vi "Start.vi"(1 "Graph refs":T2, 2 "Delays refs":T5, 6 "buttons refs":T4, 8 "error in (no error)":errorcluster, 9 "Slider cluster":T6, 10 "extra refs":T1, 11 "Control-Client in":refnum<class "Control-Client.lvclass">) -> (0 "error out":errorcluster, 3 "Control-Client out":refnum<class "Control-Client.lvclass">, 4 "Cells pos":dbl[](array[numeric]), 5 "ControlEventCom event":refnum<event-registration>)   [LabVIEW 2015, in "Control-Client.lvclass"]
uses:
  Control-Client.lvclass
  dependecies/ControlsVIs/Clusters-def/Delays-refs_CLIENT.ctl
  dependecies/ControlsVIs/Clusters-def/Controls-with-permissions_CLIENT.ctl
  controls/DigitalIndicatorELYSEpulses.ctl
  controls/CellsSD.ctl
  controls/CellBoolean.ctl
  dependecies/XControls/CellsDL/ControlDL.xctl
  controls/Gauge_pump/Gauge_pump.xctl
  controls/WCM.ctl
  dependecies/ControlsVIs/Clusters-def/Graphs_ref_Client.ctl
  dependecies/ControlsVIs/Clusters-def/graphs_TR.ctl
  dependecies/ControlsVIs/Clusters-def/Message types.ctl
  Control-Client.lvclass/Control-Client.ctl
  GeneralFunctionality/GeneralFunctionality.lvclass/GeneralFunctionality.ctl
  Message/Message.lvclass/Message.ctl
  Message/Message.lvclass
  GeneralFunctionality/GeneralFunctionality.lvclass
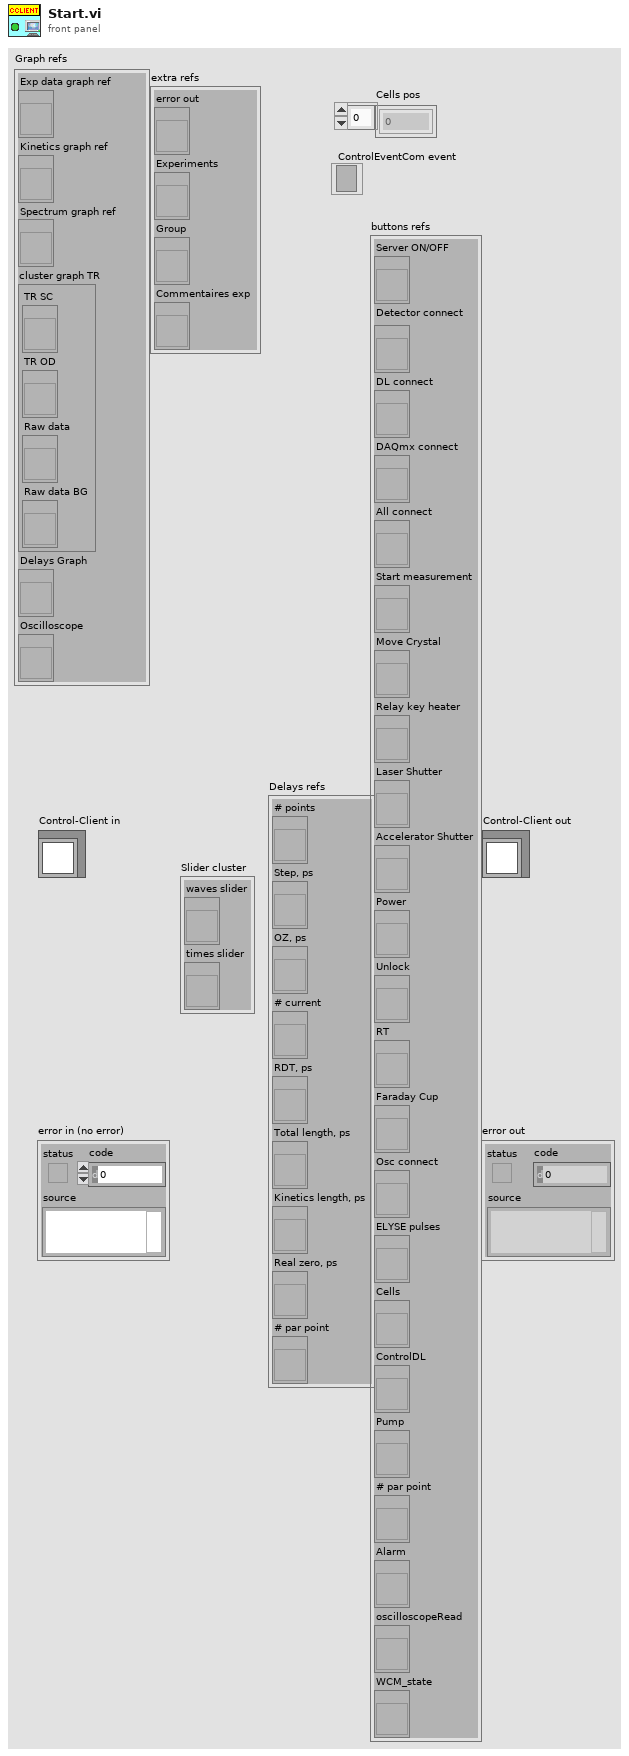
[diagram p1: front panel]
types:
  T1 = cluster{"error out":refnum<vi>, "Experiments":refnum<vi>, "Group":refnum<vi>, "Commentaires exp":refnum<vi>}
  T2 = typedef "Control-Client.lvclass/Graphs_ref_Client.ctl" = cluster{"Exp data graph ref":refnum<vi>, "Kinetics graph ref":refnum<vi>, "Spectrum graph ref":refnum<vi>, "cluster graph TR":T3, "Delays Graph":refnum<vi>, "Oscilloscope":refnum<vi>}
  T3 = typedef "graphs_TR.ctl" = cluster{"TR SC":refnum<vi>, "TR OD":refnum<vi>, "Raw data":refnum<vi>, "Raw data BG":refnum<vi>}
  T4 = typedef "Control-Client.lvclass/Controls-with-permissions_CLIENT.ctl" = cluster{"Server ON/OFF":refnum<vi>, "Detector connect":refnum<vi>, "DL connect":refnum<vi>, "DAQmx connect":refnum<vi>, "All connect":refnum<vi>, "Start measurement":refnum<vi>, "Move Crystal":refnum<vi>, "Relay key heater":refnum<vi>, "Laser Shutter":refnum<vi>, "Accelerator Shutter":refnum<vi>, "Power":refnum<vi>, "Unlock":refnum<vi>, "RT":refnum<vi>, "Faraday Cup":refnum<vi>, "Osc connect":refnum<vi>, "ELYSE pulses":refnum<vi>, "Cells":refnum<vi>, "ControlDL":refnum<vi>, "Pump":refnum<vi>, "# par point":refnum<vi>, "Alarm":refnum<vi>, "oscilloscopeRead":refnum<vi>, "WCM_state":refnum<vi>}
  T5 = typedef "Control-Client.lvclass/Delays-refs_CLIENT.ctl" = cluster{"# points":refnum<vi>, "Step, ps":refnum<vi>, "OZ, ps":refnum<vi>, "# current":refnum<vi>, "RDT, ps":refnum<vi>, "Total length, ps":refnum<vi>, "Kinetics length, ps":refnum<vi>, "Real zero, ps":refnum<vi>, "# par point":refnum<vi>}
  T6 = cluster{"waves slider":refnum<vi>, "times slider":refnum<vi>}
  T7 = typedef "Message types.ctl" = string
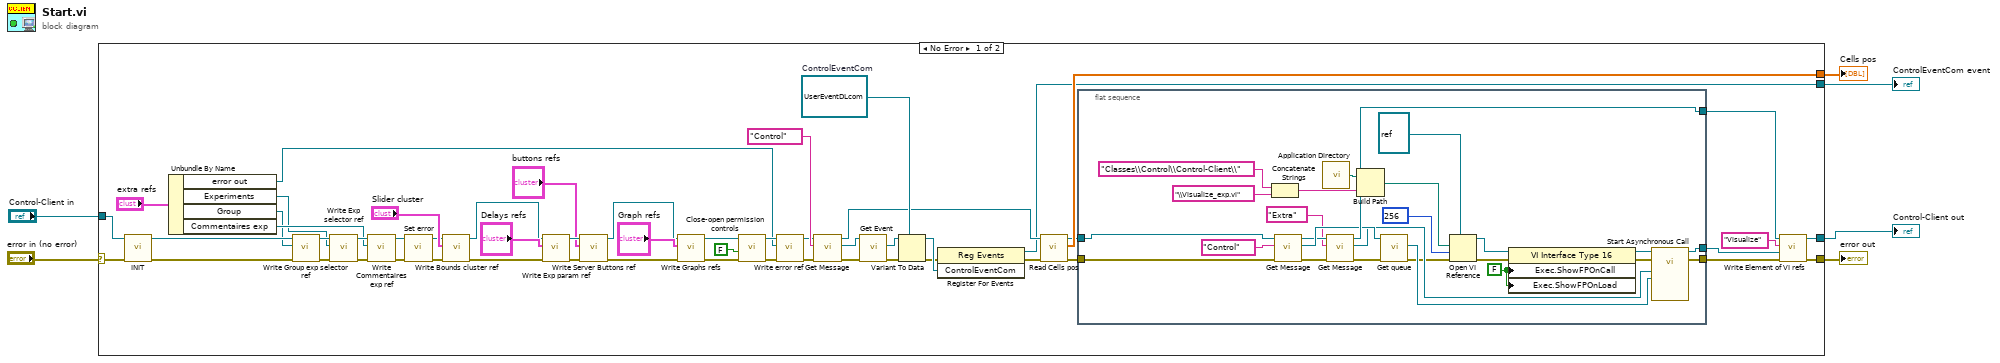
[diagram p0: block diagram]
diagram:
  n1 = case shown="No Error" "error in (no error)" {
    selector: "error in (no error)" -> [w60 w88]
    tunnel: [w16 w88] -> w5
    tunnel: [w15 w87] -> w3
    tunnel: "Control-Client in" -> [w51 w87]
    tunnel: [w18 _] -> w2
    tunnel: [w17 _] -> w1
    frame No Error {
      w26 = refnum<user-event> refnum  # ControlEventCom
      n2 = call-dynamic "INIT.vi"("error in (no error)"=w60, "Control-Client in"=w51) -> ("error out"=w59:errorcluster, "Control-Client out"=w58:refnum<class "Control-Client.lvclass">)  [unwired: 8 in]
      n3 = Unbundle By Name("extra refs") -> ("error out"=w34:refnum<vi>, "Experiments"=w31:refnum<vi>, "Group"=w32:refnum<vi>, "Commentaires exp"=w33:refnum<vi>)
      n4 = call "Write Group exp selector ref.vi"("error in (no error)"=w59, "Group exp selector ref"=w32, "Control-Client in"=w58) -> ("error out"=w56:errorcluster, "Control-Client out"=w57:refnum<class "Control-Client.lvclass">)  [unwired: 7 in]
      n5 = call "Write Exp selector ref.vi"("error in (no error)"=w56, "Exp selector ref"=w31, "Control-Client in"=w57) -> ("error out"=w55:errorcluster, "Control-Client out"=w54:refnum<class "Control-Client.lvclass">)  [unwired: 7 in]
      n6 = call "Write Commentaires exp ref.vi"("error in (no error)"=w55, "Commentaires exp"=w33, "Control-Client in"=w54) -> ("error out"=w52:errorcluster, "Control-Client out"=w53:refnum<class "Control-Client.lvclass">)  [unwired: 7 in]
      n7 = call "Set error.vi"("error in (no error)"=w52, "Control-Client in"=w53) -> ("error out"=w8:errorcluster, "Control-Client out"=w9:refnum<class "Control-Client.lvclass">)  [unwired: 8 in]
      n8 = call "Write Bounds cluster ref.vi"("error in (no error)"=w8, "Bounds cluster"="Slider cluster", "Control-Client in"=w9) -> ("error out"=w49:errorcluster, "Control-Client out"=w47:refnum<class "Control-Client.lvclass">)  [unwired: 7 in]
      n9 = call "Write Exp param ref.vi"("error in (no error)"=w49, 10:"Delays refs", "Control-Client in"=w47) -> ("error out"=w46:errorcluster, "Control-Client out"=w45:refnum<class "Control-Client.lvclass">)  [unwired: 7 in]
      n10 = call "Write Server Buttons ref.vi"("error in (no error)"=w46, "cluster of controls"="buttons refs", "Control-Client in"=w45) -> ("error out"=w43:errorcluster, "Control-Client out"=w41:refnum<class "Control-Client.lvclass">)  [unwired: 7 in]
      n11 = call "Write Graphs refs.vi"("error in (no error)"=w43, "Graph refs"="Graph refs", "Control-Client in"=w41) -> ("error out"=w39:errorcluster, "Control-Client out"=w38:refnum<class "Control-Client.lvclass">)  [unwired: 7 in]
      n12 = call "Close-open permission controls.vi"("error in (no error)"=w39, "Boolean"=FALSE, "Control-Client in"=w38) -> ("error out"=w36:errorcluster, "Control-Client out"=w37:refnum<class "Control-Client.lvclass">)  [unwired: 7 in]
      n13 = call "Write error ref.vi"("error in (no error)"=w36, "error"=w34, "GeneralFunctionality in"=w37) -> ("error out"=w23:errorcluster, "GeneralFunctionality out"=w24:refnum<class "Control-Client.lvclass">)  [unwired: 7 in]
      n14 = call "Get Message.vi"("error in (no error)"=w23, "Message type"=T7 "Control", "GeneralFunctionality en entrée"=w24) -> ("error out"=w28:errorcluster, "Message.lvclass"=w29:refnum<class "Message.lvclass">, "GeneralFunctionality en sortie"=w20:refnum<class "Control-Client.lvclass">)  [unwired: 6 in]
      n15 = call "Get Event.vi"("error in (no error)"=w28, "Message en entrée"=w29) -> ("error out"=w27:errorcluster, "UserEventCommand"=w25:refnum<user-event>)  [unwired: 7 in, 1 out]
      n16 = Variant To Data(error in=w27, type=w26, Variant=w25) -> (data=w22:refnum<user-event>, error out=w21:errorcluster)
      n17 = register-events(error in=w21, w22) -> (reference out=w17:refnum<event-registration>, error out=w19:errorcluster)  [unwired: 1 in]
      n18 = call "Read Cells pos.vi"("error in (no error)"=w19, "Control-Client in"=w20) -> ("error out"=w13:errorcluster, "Cells pos"=w18:dbl[], "Control-Client out"=w11:refnum<class "Control-Client.lvclass">)  [unwired: 7 in]
      n19 = flat-sequence {
        tunnel: w13 -> [w86]
        tunnel: [w85] -> w14
        tunnel: [w84] -> w12
        tunnel: w11 -> [w83]
        tunnel: [w82] -> w7
        frame #0 {
          w76 = FALSE ("Execution:Show Front Panel On Call")
          n20 = Concatenate Strings("Classes\\Control\\Control-Client\\" ("chaîne"), "\\Visualize_exp.vi" ("chaîne")) -> (w75:string)
          n21 = call "Get Message.vi"("error in (no error)"=w86, "Message type"=T7 "Control", "GeneralFunctionality en entrée"=w83) -> ("error out"=w67:errorcluster, "Message.lvclass"=w71:refnum<class "Message.lvclass">, "GeneralFunctionality en sortie"=w68:refnum<class "Control-Client.lvclass">)  [unwired: 6 in]
          n22 = call <vilib>:"Application Directory.vi"() -> ("Application Directory"=w80:path)
          n23 = call "Get Message.vi"("error in (no error)"=w67, "Message type"=T7 "Extra", "GeneralFunctionality en entrée"=w68) -> ("error out"=w66:errorcluster, "Message.lvclass"=w62:refnum<class "Message.lvclass">, "GeneralFunctionality en sortie"=w82:refnum<class "Control-Client.lvclass">)  [unwired: 6 in]
          n24 = Build Path(base path=w80, name or relative path=w75) -> (appended path=w81:path)
          n25 = call "Get queue.vi"("error in (no error)"=w66, "Message in"=w71) -> ("error out"=w61:errorcluster, "queue"=w70:refnum<queue>)  [unwired: 7 in, 1 out]
          n26 = Open VI Reference(type specifier VI Refnum (for type only)=refnum<vi> refnum ("spécificateur de type du refnum de VI (pour type seulement)"), vi path=w81, options=256, error in (no error)=w61) -> (vi reference=w69:refnum<vi>, error out=w77:errorcluster)  [unwired: 2 in]
          n27 = property class="VI Interface Type 16"(reference=w69, error in=w77, "Exec.ShowFPOnCall"=w76, "Exec.ShowFPOnLoad"=w76) -> (reference out=w63:refnum<vi>, error out=w64:errorcluster)
          n28 = call-by-ref "Start Asynchronous Call"(reference=w63, error in=w64, "ControlQueue"=w70, "Message in"=w62) -> (reference out=w85:refnum<vi>, error out=w84:errorcluster)  [unwired: 10 in]
        }
      }
      n29 = call "Write Element of VI refs.vi"("error in (no error)"=w12, "vi reference"=w14, "name"="Visualize", "Control-Client in"=w7) -> ("error out"=w16:errorcluster, "Control-Client out"=w15:refnum<class "Control-Client.lvclass">)  [unwired: 6 in]
    }
    frame Error {
    }
  }
  "error out" <- w5
  "Control-Client out" <- w3
  "Cells pos" <- w2
  "ControlEventCom event" <- w1
